vi "Get_last_Mod_date.vi"() -> ()   [LabVIEW 2010]
panel:
  out "Array":string[](array[string])
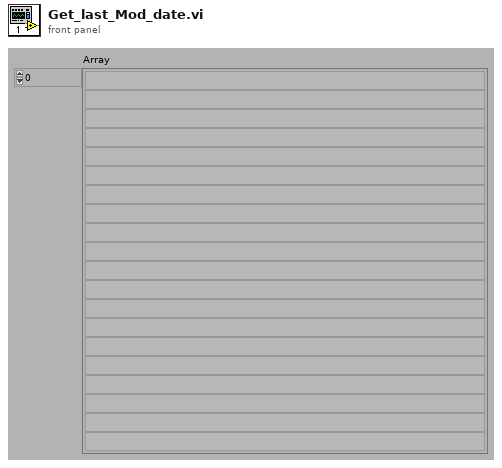
[diagram p1: front panel]
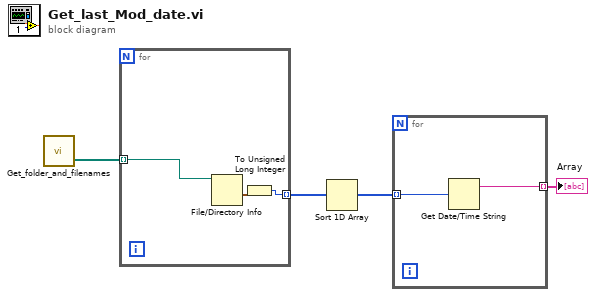
[diagram p0: block diagram]
diagram:
  n1 = call "Get_folder_and_filenames.vi"() -> ("Files"=w4:path[])  [unwired: 1 in, 1 out]
  n2 = for {
    tunnel: w4 -> [w7] mode=indexing
    tunnel: [w6] -> w3 mode=indexing
    n3 = File/Directory Info(path=w7) -> (last mod=w5:timestamp)  [unwired: 1 in, 6 out]
    n4 = To Unsigned Long Integer(number=w5) -> (unsigned 32bit integer=w6:u32)
  }
  n5 = Sort 1D Array(array=w3) -> (sorted array=w2:u32[])
  n6 = for {
    tunnel: w2 -> [w9] mode=indexing
    tunnel: [w8] -> w1 mode=indexing
    n7 = Get Date/Time String(seconds (now)=w9) -> (date string=w8:string)  [unwired: 3 out]
  }
  "Array" <- w1
